vi "Main Loop.vi"(8 "error in (no error)":errorcluster, 10 "Chart Notifier":refnum<notifier>, 11 "Message Queues":T2) -> (0 "error out":errorcluster)   [LabVIEW 2018, in "OPC UA.lvlib" / "OPC UA Module Engine.lvlib"]
uses:
  OPC UA Module Engine.lvlib
  Message Queues.ctl
  support/Message Queue/Message Cluster.ctl
  OPC Tag Data.ctl
  OPC Module Config.ctl
  Scale Module Folder/Measure Instrument/State Enum.ctl
  <vilib>/Utility/miscctls.llb/LVPoint32TypeDef.ctl
  OPC Settings.ctl
  Variable Data Cluster.ctl
  <vilib>/OPCUA/controls/NodeId.ctl
  <vilib>/OPCUA/controls/OPC UA StatusCode.ctl
  <vilib>/OPCUA/controls/Subscription ID.ctl
  <vilib>/OPCUA/controls/OPC UA Client Refnum.ctl
  <vilib>/OPCUA/controls/Subscription Data Change.ctl
  <vilib>/OPCUA/controls/Data Type.ctl
  OPC Display Cluster.ctl
  <vilib>/Platform/TimedLoop/XDataNode/timing_clust.ctl
  <vilib>/Platform/TimedLoop/XDataNode/nitl_modes.ctl
  <vilib>/Platform/TimedLoop/XDataNode/wakeup.ctl
  Tag VIs/Tag FGV Operation Enum.ctl
  support/Message Queue/Enqueue Message (Single).vi
  <vilib>/Platform/TimedLoop/XDataNode/XDataNode.xnode
  Scale Module Folder/Measure Instrument/Scale Module Engine.lvlib
  OPC UA.lvlib
  <vilib>/Platform/TimedLoop/XDataNode/XDNodeRunTimeDep.lvlib
  support/Support Library.lvlib
  Shared Variables/Dynamic Shared Variables.lvlib
  support/Message Queue/Message Queue.lvlib
panel:
  out "Tag Data 3":T1[](array[typedef])
  out "Tag Data 2":T1[](array[typedef])
  out "Tag Data Tag Names":T1[](array[typedef])
  out "Tag Data":T1[](array[typedef])
  out "Period (s)":dbl format="%_4g"
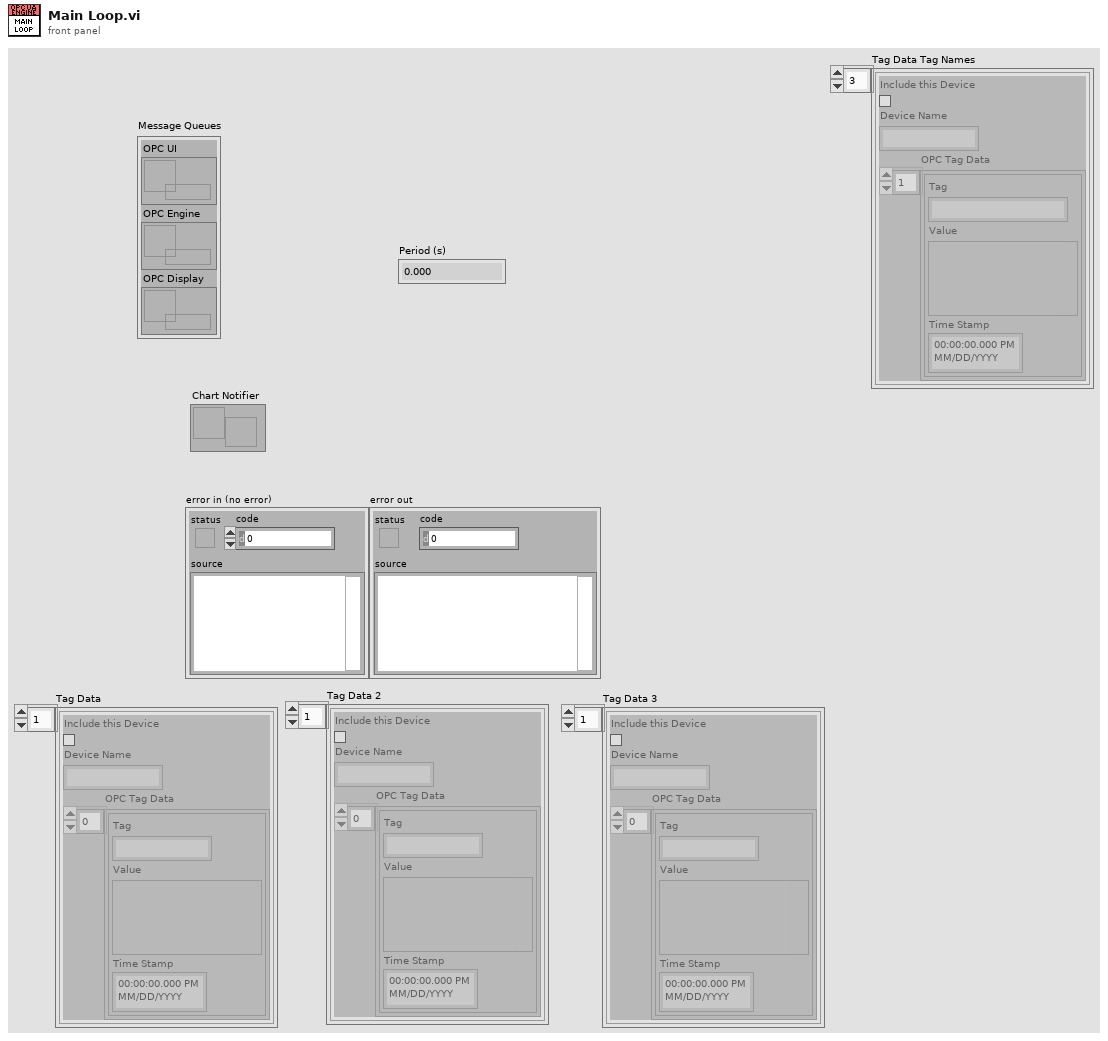
[diagram p1: front panel]
types:
  T1 = typedef "OPC UA.lvlib/OPC Tag Data.ctl" = cluster{"Include this Device":bool, "Device Name":string, "OPC Tag Data":cluster{"Tag":string, "Value":variant, "Time Stamp":timestamp}[]}
  T2 = typedef "OPC UA.lvlib/Message Queues.ctl" = cluster{"OPC UI":refnum<queue>, "OPC Engine":refnum<queue>, "OPC Display":refnum<queue>}
  T3 = typedef "OPC UA.lvlib/OPC Module Config.ctl" = cluster{"State":T4, "GUID":string, "Drop Coords":T5, "Configuration":T6, "First Iteration":bool, "Data":cluster{"Object Name":string, "Variable Array":T7[]}[], "Process Name":string, "Load Count":i32, "Log Started":bool, "subscription ID out":T10, "OPC UA client refnum out":T11, "Event Registration Refnum":refnum<event-registration>, "Start Time":timestamp, "Current Time":timestamp, "Tag Data":T1[]}
  T4 = typedef "Scale Module.lvlib/Scale Module Engine.lvlib/State Enum.ctl" = enum16{"Measuring", "Idle"}
  T5 = typedef "LVPoint32TypeDef.ctl" = cluster{"Horizontal":i32, "Vertical":i32}
  T6 = typedef "OPC UA.lvlib/OPC Settings.ctl" = cluster{"Cycle Period":dbl, "server endpoint URL":string, "security policy":cluster{"message mode":enum16{"None", "Sign", "Sign and Encrypt"}, "security":enum16{"Basic256", "Basic128Rsa15"}}, "Trust Any Server":bool}
  T7 = typedef "OPC UA.lvlib/Variable Data Cluster.ctl" = cluster{"node ID":T8, "browse name":string, "status":T9, "timestamp":timestamp, "value ":variant}
  T8 = typedef "NodeId.ctl" = string
  T9 = typedef "OPC UA StatusCode.ctl" = u32
  T10 = typedef "Subscription ID.ctl" = u32
  T11 = typedef "OPC UA Client Refnum.ctl" = refnum<k21>
  T12 = typedef "OPC UA.lvlib/OPC Display Cluster.ctl" = cluster{"URL":string, "Cycle":i32, "Updating":bool, "Tag Data":T1[]}
  T13 = typedef "XDNodeRunTimeDep.lvlib/timing_clust.ctl" = cluster{"Expected End [f-1]":u64, "Actual End [f-1]":u64, "Finished Late? [f-1]":bool, "Expected End [i-1]":u64, "Actual End [i-1]":u64, "Finished Late? [i-1]":bool, "Expected Start [i]":u64, "Actual Start [i]":u64, "Expected Start [f]":u64, "Actual Start [f]":u64, "Source Name":string, "Structure Name":string, "Period":i64, "Deadline":i64, "Offset":i64, "Start":i64, "Priority":i32, "Timeout":i32, "Mode":T14, "Wakeup Reason":T15, "Error":errorcluster, "Source Type":string, "Secondary Source Type":string, "Global End Time":u64, "Global Start Time":u64, "Frame Duration":u64, "Iteration Duration":u64, "Assigned CPU":i32, "I/O Scan Engine Mode":u32}
  T14 = typedef "XDNodeRunTimeDep.lvlib/nitl_modes.ctl" = enum32{"No Change", "Process missed periods, maintain original phase", "Discard missed periods, maintain original phase", "Process missed periods, ignore original phase", "Discard missed periods, ignore original phase"}
  T15 = typedef "XDNodeRunTimeDep.lvlib/wakeup.ctl" = enum32{"Normal", "Aborted", "Asynchronous wakeup", "Timing source error", "Timed loop error", "Timeout"}
  T16 = cluster{"enable? (F)":bool, "name":string, "alarm on":bool, "priority":u32, "ack type":enum16{"Auto", "User", "None", "Each Occurrence"}, "area":string, "description":string, "log? (T)":bool}
  T17 = typedef "Tag FGV Operation Enum.ctl" = enum16{"Init", "Set Notification Queue", "Create Tag", "Commit", "Write Tag (Numeric)", "Write Tag (Boolean)", "Read All Tags", "Read One Tag", "Delete Tag Category", "Set Alarm Parameters (Numeric)", "Set Alarm Parameters (Boolean)", "Enable All Alarms", "Disable All Alarms", "Delete All Tags", "Read Alarms", "Ack Alarm", "Read Alarm Parameters (Numeric)", "Read Alarm Parameters (Boolean)"}
  T18 = enum32{"u32BitField", "bool", "double", "string", "int8", "uint8", "int16", "uint16", "int32", "uint32", "int64", "uint64", "single", "double waveform", "int16 waveform", "array of boolean", "array of int8", "array of uint8", "array of int16", "array of uint16", "array of int32", "array of uint32", "array of int64", "array of uint64", "array of single", "array of double", "array of double waveform", "array of int16 waveform", "array of string", "variant", "timestamp", "fixed point", "custom"}
  T19 = cluster{"Tag":string, "Value":variant, "Time Stamp":timestamp}[]
  T20 = cluster{"Tag":string, "Value":variant, "Time Stamp":timestamp}
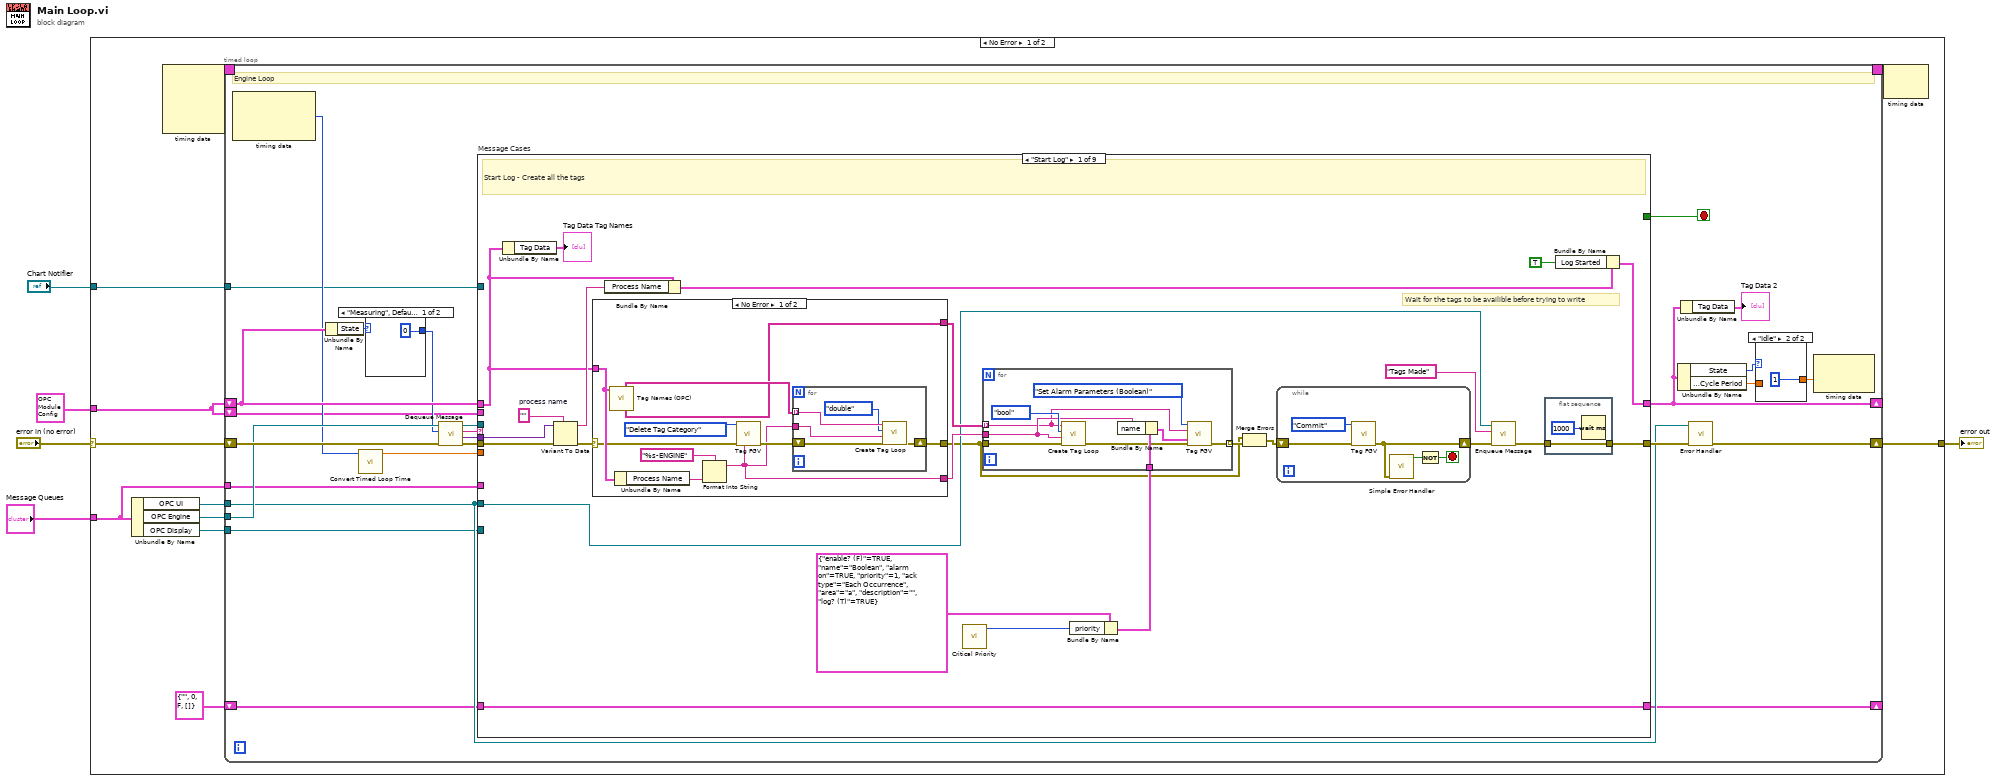
[diagram p0: block diagram]
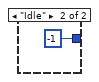
[diagram p3: hidden frame]
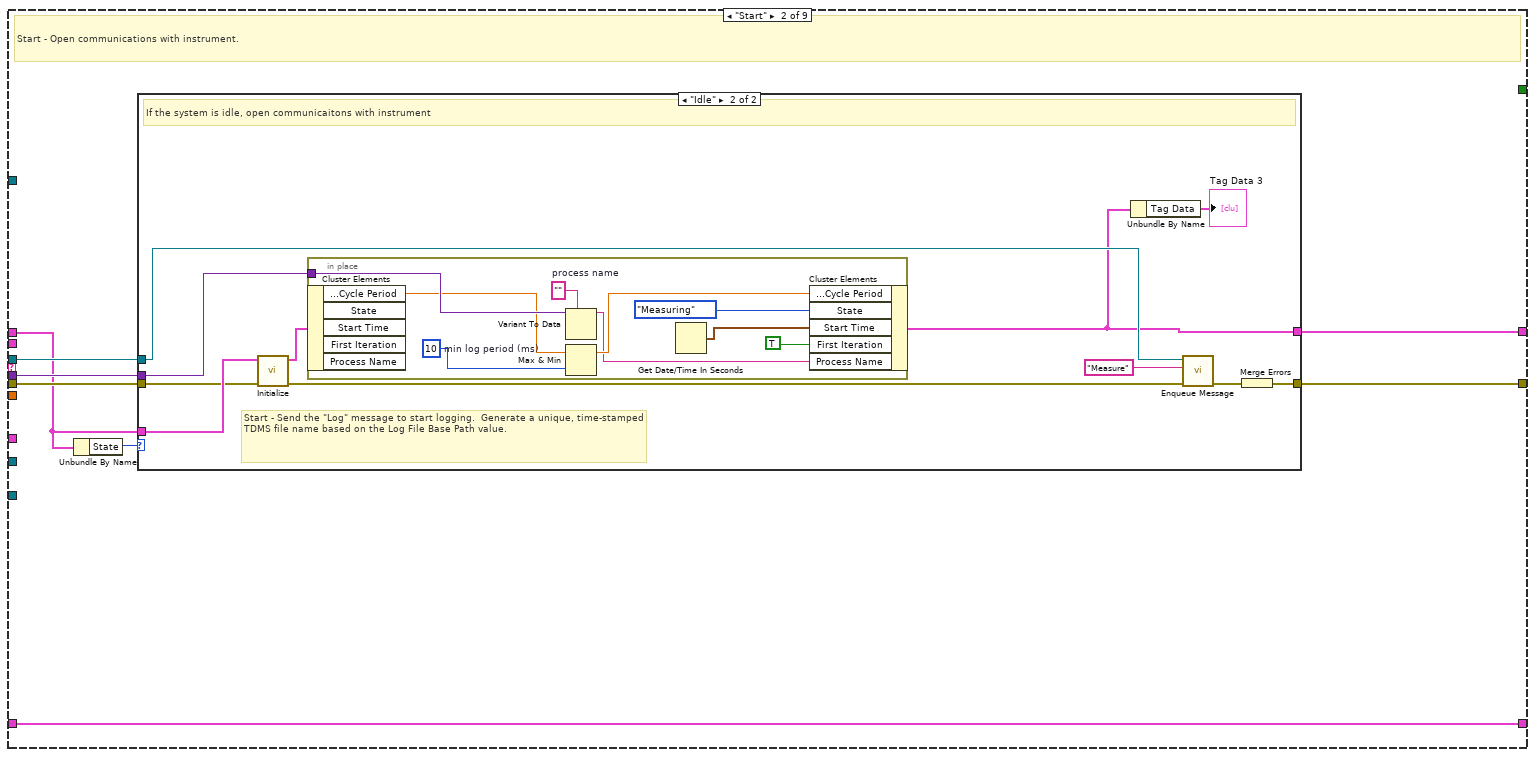
[diagram p5: hidden frame]
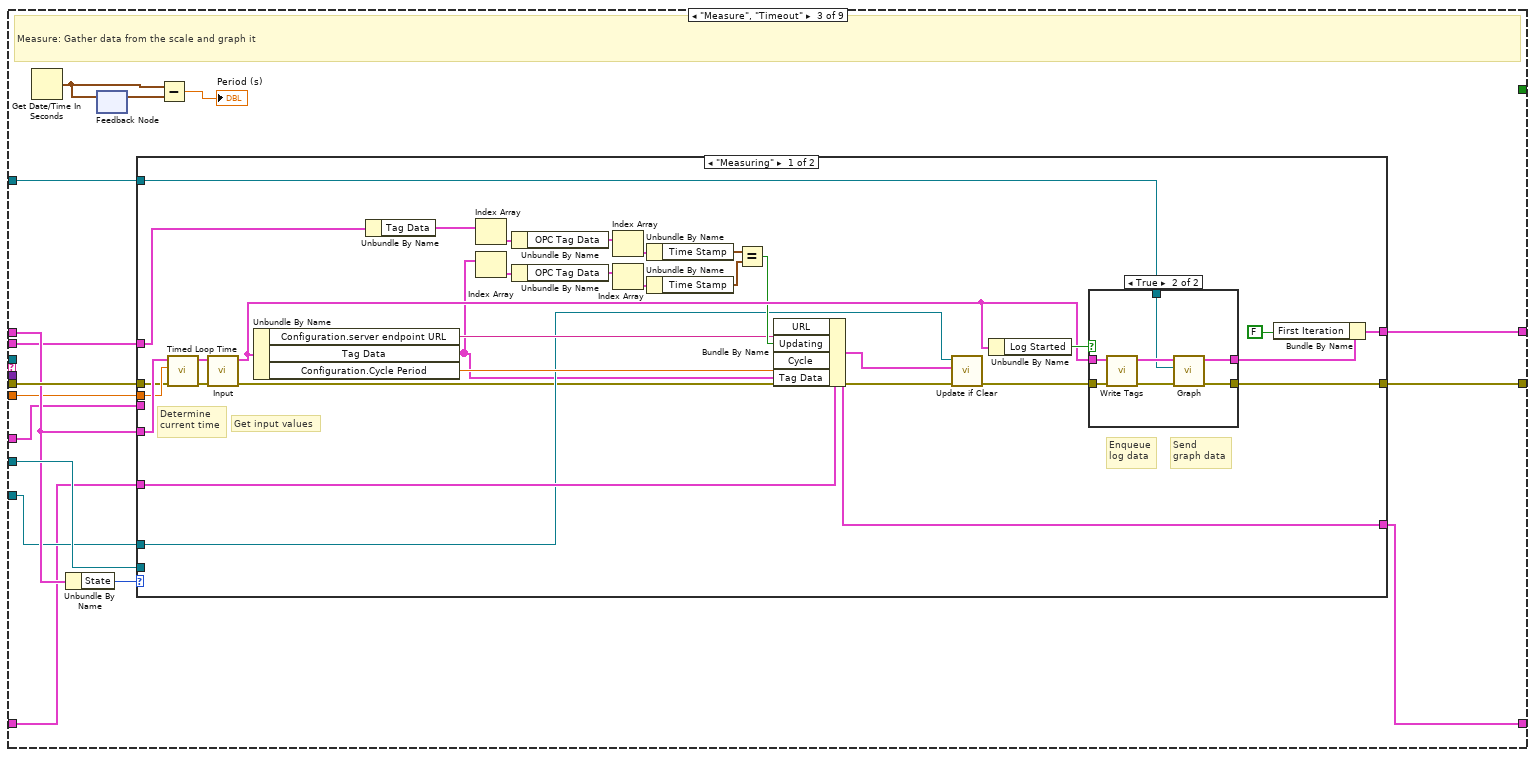
[diagram p7: hidden frame]
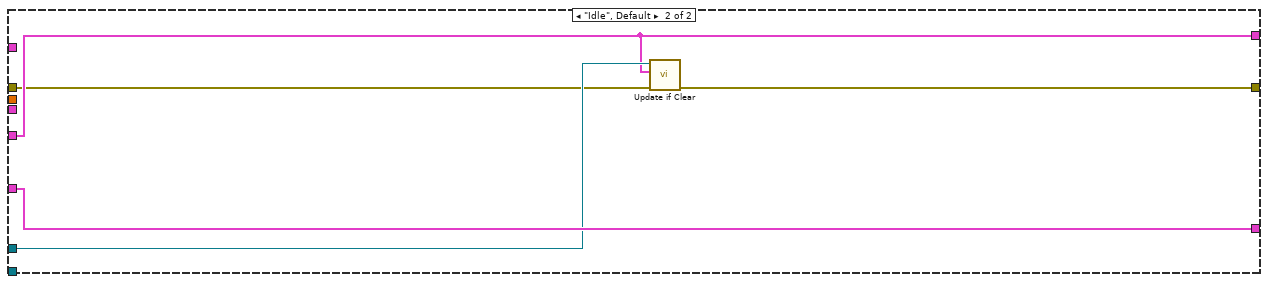
[diagram p9: hidden frame]
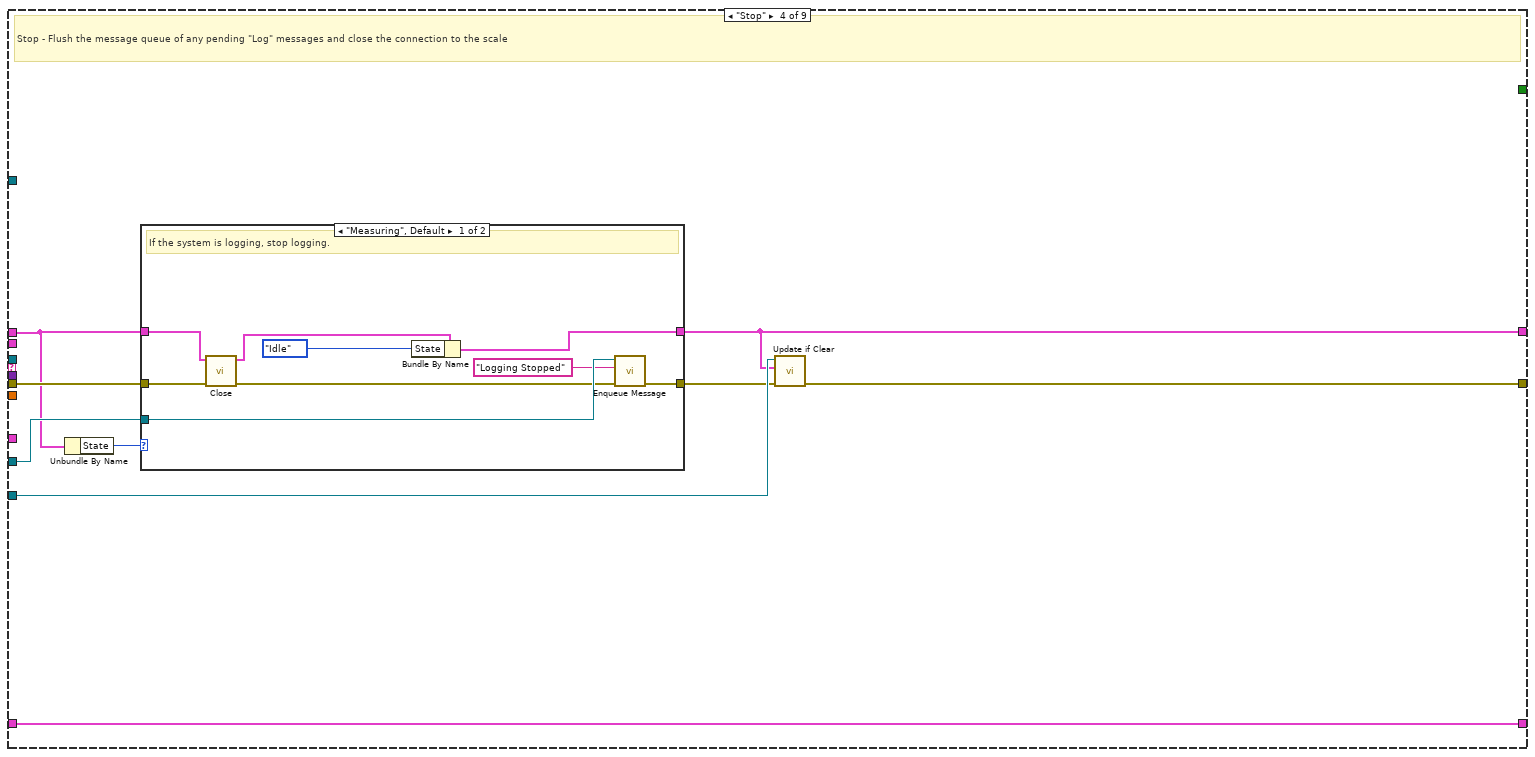
[diagram p10: hidden frame]
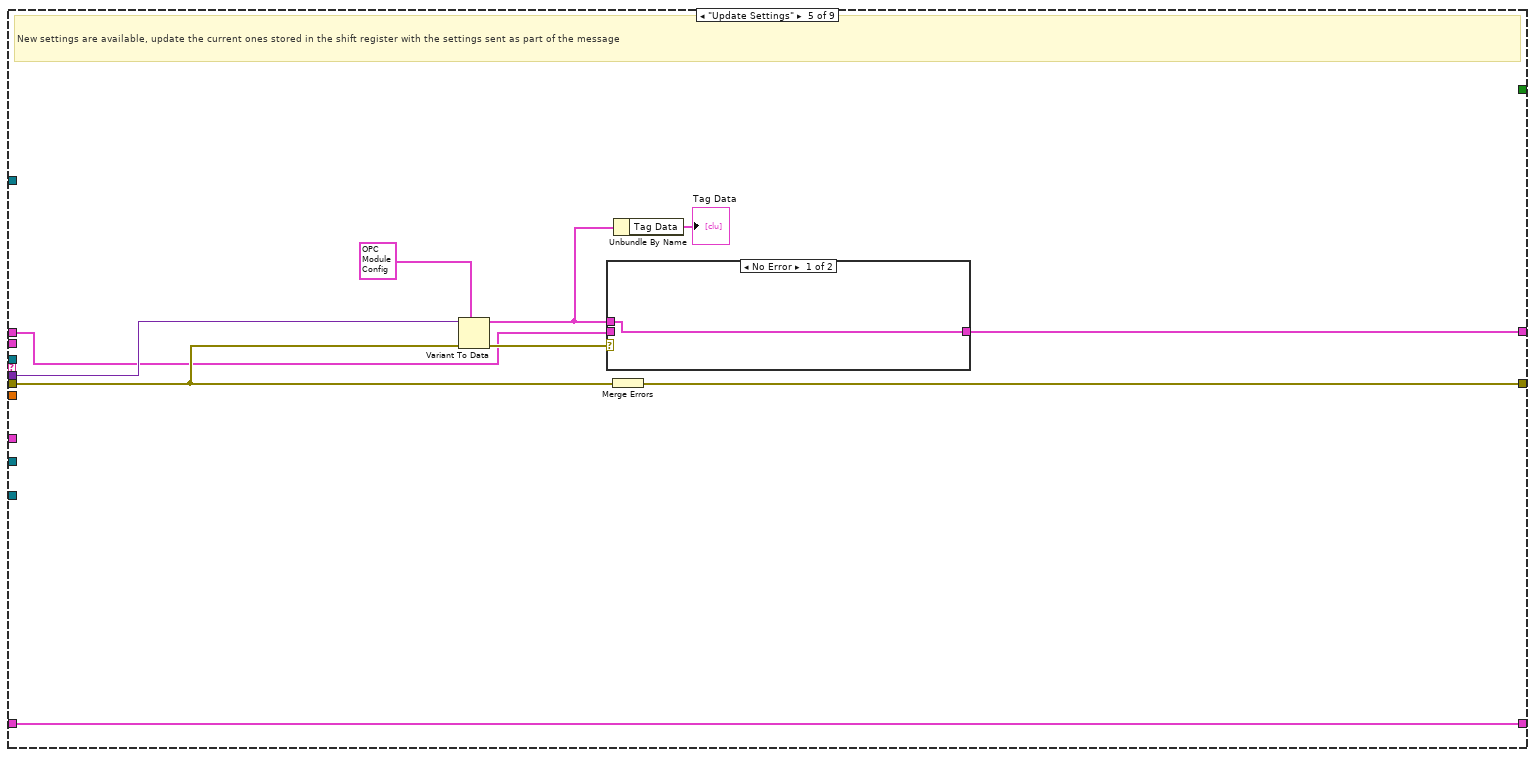
[diagram p12: hidden frame]
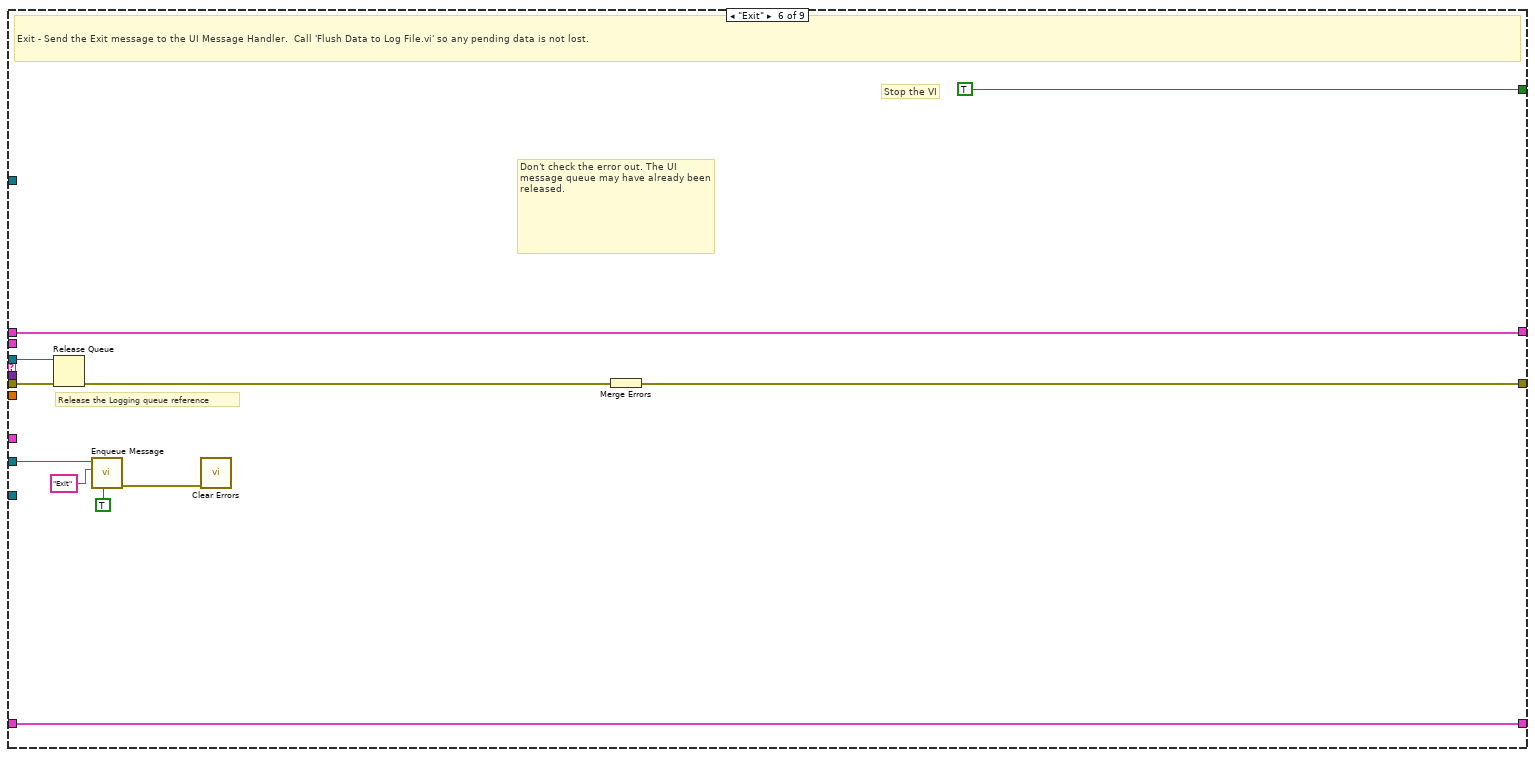
[diagram p14: hidden frame]
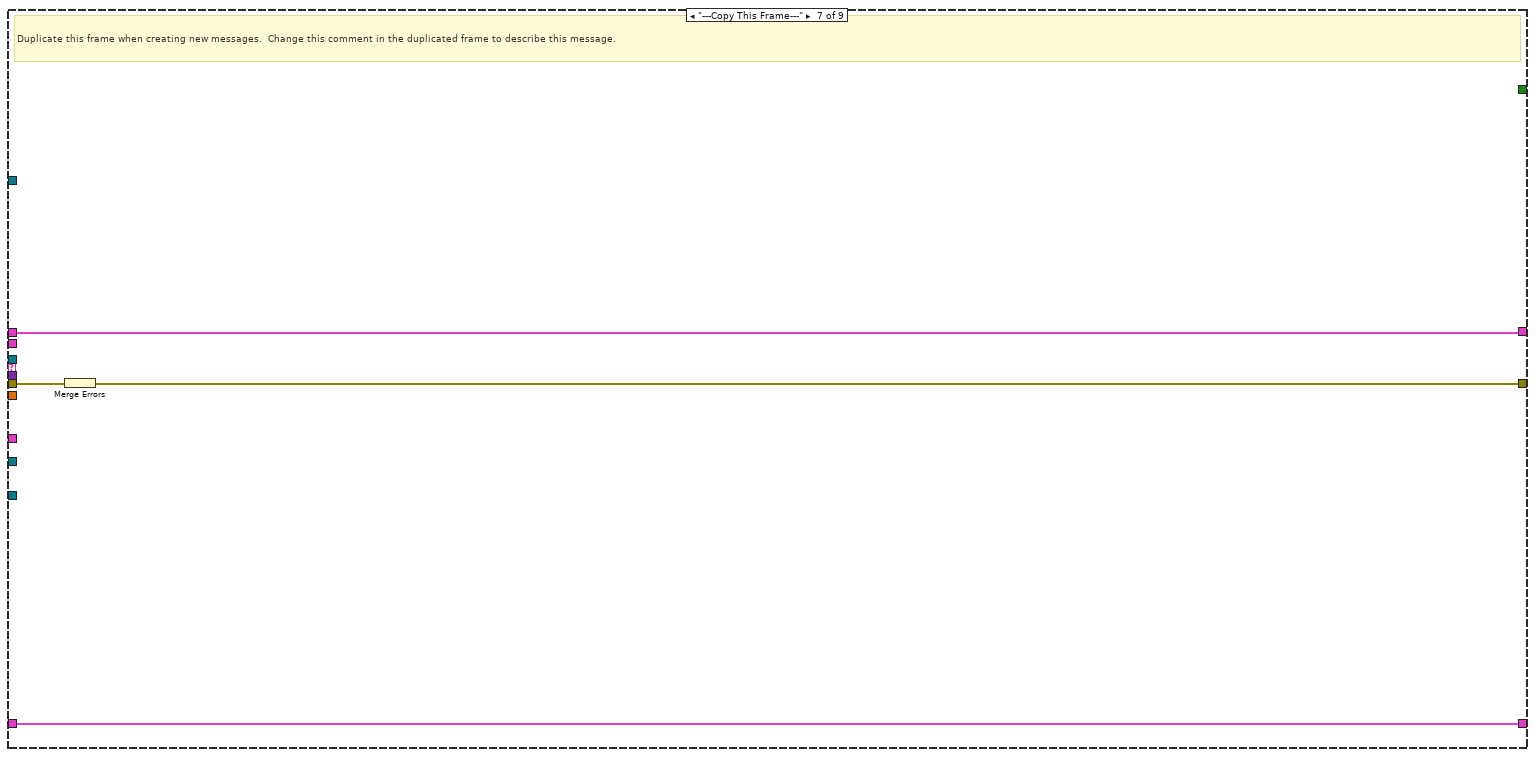
[diagram p15: hidden frame]
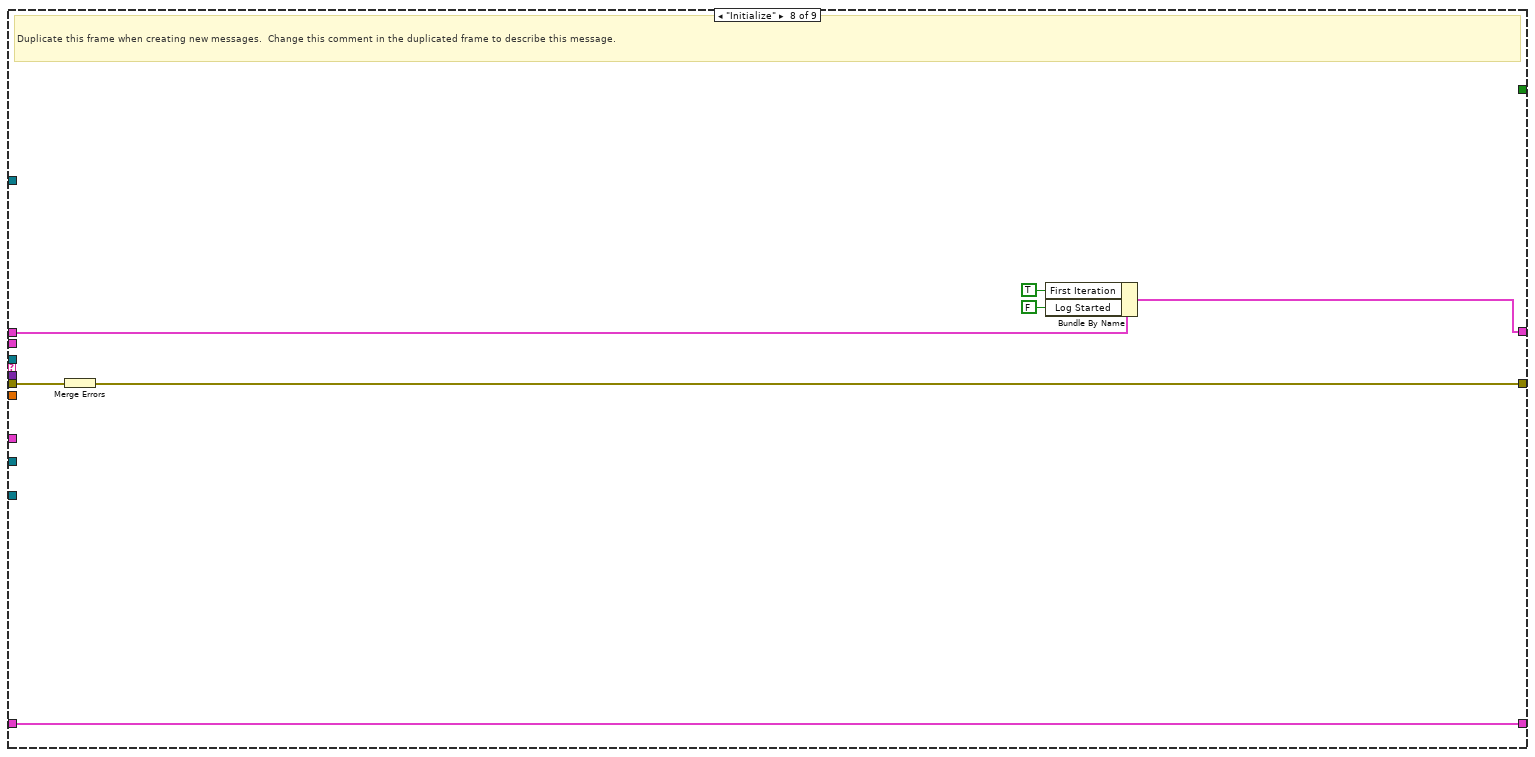
[diagram p16: hidden frame]
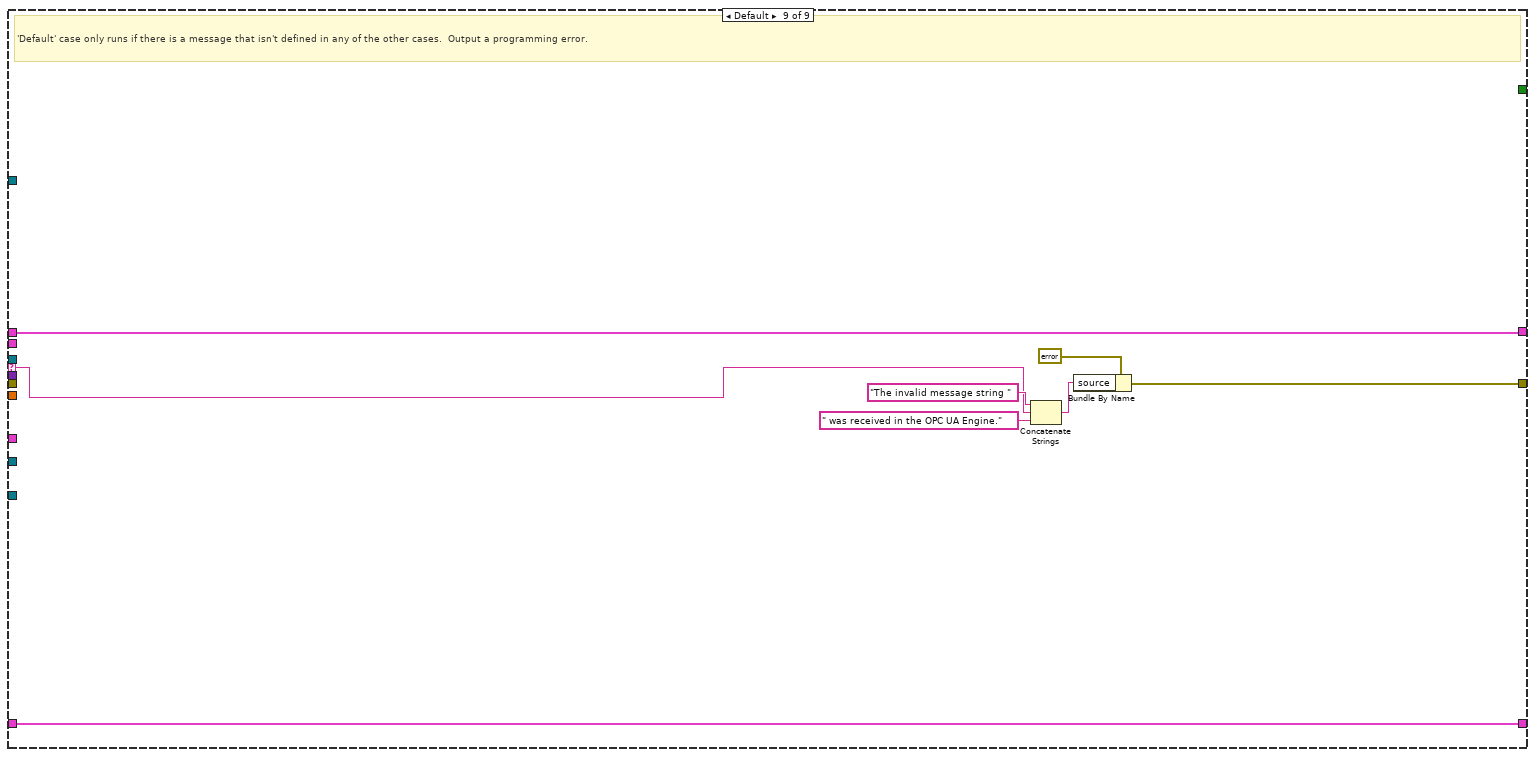
[diagram p17: hidden frame]
diagram:
  n1 = case shown="No Error" "error in (no error)" {
    selector: "error in (no error)" -> [w15 w263]
    tunnel: "Message Queues" -> [w11 _]
    tunnel: [w16 w263] -> w5
    tunnel: "Chart Notifier" -> [w9 _]
    tunnel: T3 {"State"=enum."Idle", "GUID"="", "Drop Coords"={"Horizontal"=0, "Vertical"=0}, "Configuration"={"Cycle Period"=500.0, "server endpoint URL"="opc.tcp://10.131.1.22:4840", "security policy"={"message mode"=enum."None", "security"=enum."Basic256"}, "Trust Any Server"=FALSE}, "First Iteration"=FALSE, "Data"=[], "Process Name"="", "Load Count"=0, "Log Started"=FALSE, "subscription ID out"=0, "OPC UA client refnum out"="", "Event Registration Refnum"=refnum, "Start Time"=timestamp(0 s since 1904-01-01), "Current Time"=timestamp(0 s since 1904-01-01), "Tag Data"=[]} ("OPC Module Config") -> [w6 _]
    frame No Error {
      n2 = Unbundle By Name(w11) -> ("OPC UI"=w14:refnum<queue>, "OPC Engine"=w10:refnum<queue>, "OPC Display"=w8:refnum<queue>)
      n3 = node-c288() -> (w13:T13)  [unwired: 4 in]
      n4 = timed-loop {
        tunnel: w10 -> [w36]
        shift-right: [w18] -> _
        shift-left: w6 -> [w32]
        shift-right: [w34] -> w16
        shift-left: w15 -> [w41]
        tunnel: w14 -> [w33]
        timing: w13 -> [_]
        timing-out: [_] -> w12
        tunnel: w11 -> [w24]
        tunnel: w9 -> [w23]
        tunnel: w8 -> [w22]
        shift-right: [w21] -> _
        shift-left: T12 {"URL"="", "Cycle"=0, "Updating"=FALSE, "Tag Data"=[]} ("OPC Display Cluster") -> [w20]
        shift-left: w6 -> [w19]
        stop <- w42 stop-if-true
        # "Engine Loop"
        n5 = node-c288() -> (w26:i64)  [unwired: 1 in, 2 out]
        n6 = Unbundle By Name(w32) -> ("State"=w31:T4)
        n7 = call "Convert Timed Loop Time.vi"("Actual Start [i]"=w26) -> ("ET since start (s)"=w25:dbl)  [unwired: 10 in]
        n8 = case shown="\"Measuring\", Default" w31 {
          tunnel: [0 ("timeout in ms (-1)") -1 ("timeout in ms (-1)")] -> w30
          frame "Measuring", Default {
          }
          frame "Idle" {
          }
        }
        n9 = call "Dequeue Message.vi"("error in (no error)"=w41, "timeout in ms (-1)"=w30, "Message Queue"=w36) -> ("error out"=w40:errorcluster, "Message Data"=w38:variant, "Message"=w39:string, "dup Message Queue"=w37:refnum<queue>)  [unwired: 5 in]
        n10 = case "Message Cases" shown="\"Start Log\"" w39 {
          selector: w39 -> [_ _ _ _ _ _ _ _ w254]
          tunnel: w37 -> [_ w114 _ _ _ w235 _ _ _]
          tunnel: w40 -> [w70 w113 w150 w207 w226 w238 w245 w252 _]
          tunnel: [w55 w115 w151 w199 w228 w240 w244 w251 w253] -> w35
          tunnel: w32 -> [w53 w110 w149 w204 w224 w231 w242 w249 w259]
          tunnel: [_ _ _ _ _ TRUE _ _ _] -> w42
          tunnel: w38 -> [w71 w111 _ _ w227 _ _ _ _]
          tunnel: w33 -> [w59 _ w152 w206 _ w239 _ _ _]
          tunnel: w25 -> [_ _ w148 _ _ _ _ _ _]
          tunnel: w24 -> [_ _ w147 _ _ _ _ _ _]
          tunnel: w23 -> [_ _ w143 _ _ _ _ _ _]
          tunnel: w22 -> [_ _ w142 w202 _ _ _ _ _]
          tunnel: w20 -> [w75 w109 w141 w203 w223 w232 w243 w250 w260]
          tunnel: [w75 w109 w140 w203 w223 w232 w243 w250 w260] -> w21
          tunnel: [w62 w108 w138 w201 w222 w231 w242 w246 w259] -> w18
          tunnel: w19 -> [_ _ w139 _ _ _ _ _ _]
          frame "Start Log" {
            w74 = ""  # process name
            # "Wait for the tags to be availible before trying to write"
            # "Start Log - Create all the tags"
            n11 = Unbundle By Name(w53) -> ("Tag Data"=→"Tag Data Tag Names":T1[])
            n12 = Variant To Data(error in=w70, type=w74, Variant=w71) -> (data=w72:string, error out=w73:errorcluster)
            n13 = case shown="No Error" w73 {
              selector: w73 -> [w94 w107]
              tunnel: [w101 w107] -> w54
              tunnel: [w92 _] -> w66
              tunnel: [w98 _] -> w65
              tunnel: w53 -> [w97 _]
              frame No Error {
                n14 = call "Tag Names (OPC).vi"("OPC Module Config"=w97) -> ("All Boolean Tags"=w98:string[], "All  Numeric Tags"=w99:string[])  [unwired: 8 in, 1 out]
                n15 = Unbundle By Name(w97) -> ("Process Name"=w96:string)
                n16 = Format Into String(format string="%s-ENGINE", w96) -> (resulting string=w92:string)  [unwired: 2 in, 1 out]
                n17 = call "Tag FGV.vi"("Operation"=Tag_FGV_Operation_Enum."Delete Tag Category", "error in (no error)"=w94, "Tag Category"=w92) -> ("error out"=w93:errorcluster)  [unwired: 5 in, 7 out]
                n18 = for {
                  shift-right: [w106] -> w101
                  shift-left: w93 -> [w105]
                  tunnel: w92 -> [w102]
                  tunnel: w99 -> [w104] mode=indexing
                  n19 = call "Create Tag Loop.vi"("error in (no error)"=w105, "Tag Category"=w102, "data type"=T18."double", "Tag Name"=w104) -> ("error out"=w106:errorcluster)  [unwired: 7 in]
                }
              }
              frame Error {
              }
            }
            n20 = Bundle By Name(cluster=w53, "Process Name"=w72) -> (w63:T3)
            n21 = call "Critical Priority.vi"() -> ("critical priority"=w68:i32)  [unwired: 11 in]
            n22 = Bundle By Name(cluster=T16 {"enable? (F)"=TRUE, "name"="Boolean", "alarm on"=TRUE, "priority"=1, "ack type"=enum."Each Occurrence", "area"="a", "description"="", "log? (T)"=TRUE} ("Boolean alarm settings"), "priority"=w68) -> (w67:T16)
            n23 = for {
              tunnel: w67 -> [w91]
              tunnel: [w83] -> w64 mode=indexing
              tunnel: w65 -> [w86] mode=indexing
              tunnel: w66 -> [w88]
              tunnel: w54 -> [w90]
              n24 = call "Create Tag Loop.vi"("error in (no error)"=w90, "Tag Category"=w88, "data type"=T18."bool", "Tag Name"=w86) -> ("error out"=w84:errorcluster)  [unwired: 7 in]
              n25 = Bundle By Name(cluster=w91, "name"=w88) -> (w85:T16)
              n26 = call "Tag FGV.vi"("Operation"=Tag_FGV_Operation_Enum."Set Alarm Parameters (Boolean)", "Tag Name"=w86, "Data"=w85, "error in (no error)"=w84) -> ("error out"=w83:errorcluster)  [unwired: 4 in, 7 out]
            }
            n27 = Merge Errors(w54, w64) -> (w57:errorcluster)
            n28 = while {
              shift-right: [w78] -> w58
              shift-left: w57 -> [w79]
              stop <- w81 stop-if-true
              n29 = call "Tag FGV.vi"("Operation"=Tag_FGV_Operation_Enum."Commit", "error in (no error)"=w79) -> ("error out"=w78:errorcluster)  [unwired: 6 in, 7 out]
              n30 = call <vilib>:"Simple Error Handler.vi"("error in (no error)"=w78) -> ("error?"=w82:bool)  [unwired: 4 in, 4 out]
              n31 = Not(x=w82) -> (.not. x?=w81:bool)
            }
            n32 = call-poly "Enqueue Message.vi"("error in (no error)"=w58, "Message"="Tags Made", "Message Queue"=w59) -> ("error out"=w56:errorcluster)  [unwired: 7 in, 1 out]
            n33 = flat-sequence {
              tunnel: [w76] -> w55
              tunnel: w56 -> [w76]
              frame #0 {
                n34 = Wait (ms)(milliseconds to wait=u32 1000) -> ()  [unwired: 1 out]
              }
            }
            n35 = Bundle By Name(cluster=w63, "Log Started"=TRUE) -> (w62:T3)
          }
          frame "Start" {
            # "Start - Open communications with instrument."
            n36 = Unbundle By Name(w110) -> ("State"=w112:T4)
            n37 = case shown="\"Idle\"" w112 {
              tunnel: [w116 w128] -> w115
              tunnel: w114 -> [_ w125]
              tunnel: w113 -> [w116 w122]
              tunnel: w110 -> [w117 w123]
              tunnel: [w117 w118] -> w108
              tunnel: w111 -> [_ w124]
              frame "Measuring", Default {
                # "The system is already running. Ignore the \"Start\" message."
              }
              frame "Idle" {
                # "Start - Send the \"Log\" message to start logging.  Generate a unique, time-stamped TDMS file name based on the Log File Base Path value."
                # "If the system is idle, open communicaitons with instrument"
                n38 = call "Initialize.vi"("error in"=w122, "OPC Module Config In"=w123) -> ("error out"=w121:errorcluster, "OPC Module Config Out"=w120:T3)  [unwired: 8 in]
                n39 = in-place {
                  in-place-border: w124 -> [w135]
                  w136 = ""  # process name
                  w137 = 10  # min log period (ms)
                  n40 = in-place-cluster #1(w120) -> ("Configuration.Cycle Period"=w134:dbl)  [unwired: 4 out]
                  n41 = Variant To Data(type=w136, Variant=w135) -> (data=w129:string)  [unwired: 1 in, 1 out]
                  n42 = Max & Min(x=w134, y=w137) -> (max(x,y)=w133:dbl)  [unwired: 1 out]
                  n43 = Get Date/Time In Seconds() -> (seconds since 1Jan1904=w131:timestamp)
                  n44 = in-place-cluster #1("Configuration.Cycle Period"=w133, "State"=State_Enum."Measuring", "Start Time"=w131, "First Iteration"=TRUE, "Process Name"=w129) -> (w118:T3)
                }
                n45 = Unbundle By Name(w118) -> ("Tag Data"=→"Tag Data 3":T1[])
                n46 = call-poly "Enqueue Message.vi"("error in (no error)"=w121, "Message"="Measure", "Message Queue"=w125) -> ("error out"=w126:errorcluster)  [unwired: 7 in, 1 out]
                n47 = Merge Errors(w126) -> (w128:errorcluster)
              }
            }
          }
          frame "Measure", "Timeout" {
            # "Measure: Gather data from the scale and graph it"
            n48 = Get Date/Time In Seconds() -> (seconds since 1Jan1904=w145:timestamp)
            n49 = Unbundle By Name(w149) -> ("State"=w153:T4)
            n50 = feedback-in #2(w145) -> ()
            n51 = feedback #2() -> (w146:timestamp)  [unwired: 1 in]
            n52 = case shown="\"Measuring\"" w153 {
              tunnel: w150 -> [w174 w195]
              tunnel: w149 -> [w176 w196]
              tunnel: w152 -> [_ _]
              tunnel: [w184 w194] -> w151
              tunnel: [w182 w196] -> w138
              tunnel: w148 -> [w175 _]
              tunnel: w147 -> [_ _]
              tunnel: w143 -> [w180 _]
              tunnel: w142 -> [w158 w197]
              tunnel: w141 -> [w179 w198]
              tunnel: [w157 w198] -> w140
              tunnel: w139 -> [w170 _]
              frame "Measuring" {
                # "Determine\ncurrent time"
                # "Send\ngraph data"
                # "Enqueue\nlog data"
                # "Get input values"
                n53 = call "Timed Loop Time.vi"("error in (no error)"=w174, "ET since start (s)"=w175, "OPC Module Config In"=w176) -> ("error out"=w172:errorcluster, "OPC Module Config Out"=w173:T3)  [unwired: 7 in]
                n54 = call "Input.vi"("error in"=w172, "OPC Module Config In"=w173) -> ("error out"=w156:errorcluster, "OPC Module Config Out"=w171:T3)  [unwired: 8 in]
                n55 = Unbundle By Name(w171) -> ("Configuration.server endpoint URL"=w159:string, "Tag Data"=w154:T1[], "Configuration.Cycle Period"=w178:dbl)
                n56 = Unbundle By Name(w170) -> ("Tag Data"=w169:T1[])
                n57 = Index Array(array=w169) -> (element=w168:T1)  [unwired: 1 in]
                n58 = Index Array(array=w154) -> (element=w163:T1)  [unwired: 1 in]
                n59 = Unbundle By Name(w168) -> ("OPC Tag Data"=w167:T19)
                n60 = Unbundle By Name(w163) -> ("OPC Tag Data"=w164:T19)
                n61 = Index Array(array=w167) -> (element=w166:T20)  [unwired: 1 in]
                n62 = Index Array(array=w164) -> (element=w165:T20)  [unwired: 1 in]
                n63 = Unbundle By Name(w166) -> ("Time Stamp"=w162:timestamp)
                n64 = Unbundle By Name(w165) -> ("Time Stamp"=w161:timestamp)
                n65 = Equal?(x=w162, y=w161) -> (x = y?=w160:bool)
                n66 = Bundle By Name(cluster=w179, "URL"=w159, "Updating"=w160, "Cycle"=w178, "Tag Data"=w154) -> (w157:T12)
                n67 = call "Update if Clear.vi"("error in (no error)"=w156, "Message Data"=w157, "Queue in"=w158) -> ("error out"=w155:errorcluster)  [unwired: 8 in]
                n68 = Unbundle By Name(w171) -> ("Log Started"=w177:bool)
                n69 = case shown="True" w177 {
                  tunnel: [w185 w187] -> w184
                  tunnel: [w186 w188] -> w183
                  tunnel: w180 -> [_ w190]
                  tunnel: w171 -> [w186 w193]
                  tunnel: w155 -> [w185 w192]
                  frame False {
                  }
                  frame True {
                    n70 = call "Write Tags.vi"("error in (no error)"=w192, "OPC Module Config In"=w193) -> ("error out"=w189:errorcluster, "OPC Module Config Out"=w191:T3)  [unwired: 8 in]
                    n71 = call "Graph.vi"("error in (no error)"=w189, "notifier out"=w190, "OPC Module Config In"=w191) -> ("error out"=w187:errorcluster, "OPC Module Config Out"=w188:T3)  [unwired: 7 in]
                  }
                }
                n72 = Bundle By Name(cluster=w183, "First Iteration"=FALSE) -> (w182:T3)
              }
              frame "Idle", Default {
                n73 = call "Update if Clear.vi"("error in (no error)"=w195, "Message Data"=w196, "Queue in"=w197) -> ("error out"=w194:errorcluster)  [unwired: 8 in]
              }
            }
            n74 = Subtract(x=w145, y=w146) -> (x-y=→"Period (s)":dbl)
          }
          frame "Stop" {
            # "Stop - Flush the message queue of any pending \"Log\" messages and close the connection to the scale"
            n75 = Unbundle By Name(w204) -> ("State"=w205:T4)
            n76 = case shown="\"Measuring\", Default" w205 {
              tunnel: [w212 w218] -> w200
              tunnel: w207 -> [w210 w218]
              tunnel: w206 -> [w216 _]
              tunnel: w204 -> [w211 w217]
              tunnel: [w214 w217] -> w201
              frame "Measuring", Default {
                # "If the system is logging, stop logging."
                n77 = call "Close.vi"("error in"=w210, "OPC Module Config In"=w211) -> ("error out"=w208:errorcluster, "OPC Module Config Out"=w209:T3)  [unwired: 8 in]
                n78 = Bundle By Name(cluster=w209, "State"=State_Enum."Idle") -> (w214:T3)
                n79 = call-poly "Enqueue Message.vi"("error in (no error)"=w208, "Message"="Logging Stopped", "Message Queue"=w216) -> ("error out"=w212:errorcluster)  [unwired: 7 in, 1 out]
              }
              frame "Idle" {
                # "The system is already idle. Ignore the \"Stop\" message."
              }
            }
            n80 = call "Update if Clear.vi"("error in (no error)"=w200, "Message Data"=w201, "Queue in"=w202) -> ("error out"=w199:errorcluster)  [unwired: 8 in]
          }
          frame "Update Settings" {
            # "New settings are available, update the current ones stored in the shift register with the settings sent as part of the message"
            n81 = Variant To Data(error in=w226, type=T3 {"State"=enum."Idle", "GUID"="", "Drop Coords"={"Horizontal"=0, "Vertical"=0}, "Configuration"={"Cycle Period"=500.0, "server endpoint URL"="opc.tcp://10.131.1.22:4840", "security policy"={"message mode"=enum."None", "security"=enum."Basic256"}, "Trust Any Server"=FALSE}, "First Iteration"=FALSE, "Data"=[], "Process Name"="", "Load Count"=0, "Log Started"=FALSE, "subscription ID out"=0, "OPC UA client refnum out"="", "Event Registration Refnum"=refnum, "Start Time"=timestamp(0 s since 1904-01-01), "Current Time"=timestamp(0 s since 1904-01-01), "Tag Data"=[]} ("OPC Module Config"), Variant=w227) -> (data=w219:T3, error out=w225:errorcluster)
            n82 = case shown="No Error" w225 {
              tunnel: w224 -> [_ _]
              tunnel: w219 -> [w229 w230]
              tunnel: [w229 w230] -> w222
              frame No Error {
              }
              frame Error {
              }
            }
            n83 = Merge Errors(w226) -> (w228:errorcluster)
            n84 = Unbundle By Name(w219) -> ("Tag Data"=→"Tag Data":T1[])
          }
          frame "Exit" {
            # "Release the Logging queue reference"
            # "Don't check the error out. The UI message queue may have already been released."
            # "Stop the VI"
            # "Exit - Send the Exit message to the UI Message Handler.  Call 'Flush Data to Log File.vi' so any pending data is not lost."
            n85 = Release Queue(queue=w235, error in (no error)=w238) -> (error out=w234:errorcluster)  [unwired: 1 in, 2 out]
            n86 = call-poly "Enqueue Message.vi"("Priority Message? (F)"=TRUE, "Message"="Exit", "Message Queue"=w239) -> ("error out"=w233:errorcluster)  [unwired: 7 in, 1 out]
            n87 = call <vilib>:"Clear Errors.vi"("error in (no error)"=w233) -> ()  [unwired: 5 in, 2 out]
            n88 = Merge Errors(w234) -> (w240:errorcluster)
          }
          frame "---Copy This Frame---" {
            # "Duplicate this frame when creating new messages.  Change this comment in the duplicated frame to describe this message."
            n89 = Merge Errors(w245) -> (w244:errorcluster)
          }
          frame "Initialize" {
            # "Duplicate this frame when creating new messages.  Change this comment in the duplicated frame to describe this message."
            n90 = Merge Errors(w252) -> (w251:errorcluster)
            n91 = Bundle By Name(cluster=w249, "First Iteration"=TRUE, "Log Started"=FALSE) -> (w246:T3)
          }
          frame Default {
            # "'Default' case only runs if there is a message that isn't defined in any of the other cases.  Output a programming error."
            n92 = Concatenate Strings("The invalid message string " ("string"), w254, " was received in the OPC UA Engine." ("string")) -> (w255:string)
            n93 = Bundle By Name(cluster=errorcluster {"status"=TRUE, "code"=1, "source"=""} ("error constant"), "source"=w255) -> (w253:errorcluster)
          }
        }
        n94 = Unbundle By Name(w18) -> ("State"=w29:T4, "Configuration.Cycle Period"=w27:dbl)
        n95 = Unbundle By Name(w18) -> ("Tag Data"=→"Tag Data 2":T1[])
        n96 = call "Error Handler.vi"("error in (no error)"=w35, "Message Queue"=w33) -> ("dup error in"=w34:errorcluster)  [unwired: 8 in, 1 out]
        n97 = case shown="\"Idle\"" w29 {
          tunnel: [w43 1] -> w28
          tunnel: w27 -> [w43 _]
          frame "Measuring" {
          }
          frame "Idle" {
          }
        }
        n98 = node-c288(w28) -> ()  [unwired: 1 in, 1 out]
      }
      n99 = node-c288(w12) -> ()  [unwired: 1 out]
    }
    frame Error {
    }
  }
  "error out" <- w5
